vi "Read Value (variant).vi"(8 "error in (no error)":errorcluster, 11 "Bool D Element in":refnum<class "Bool D Element.lvclass">) -> (0 "error out":errorcluster, 2 "Variant":variant, 3 "Bool D Element out":refnum<class "Bool D Element.lvclass">)   [LabVIEW 2018, in "D Datagrid Library.lvlib" / "Bool D Element.lvclass"]
uses:
  Bool D Element.lvclass
  Bool D Element.lvclass/Bool D Element.ctl
  Read Value.vi
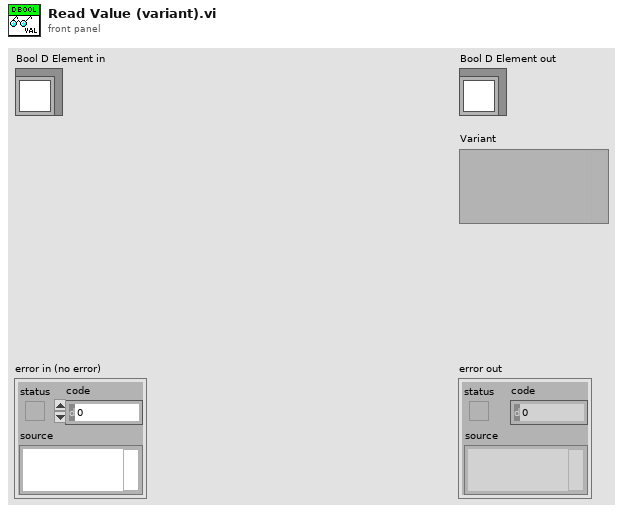
[diagram p1: front panel]
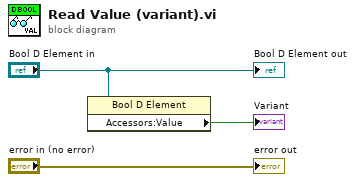
[diagram p0: block diagram]
diagram:
  n1 = property class="Bool D Element"(reference="Bool D Element in") -> ("Accessors:Value"=→"Variant":bool)  [unwired: 1 in, 2 out]
  "error out" <- "error in (no error)"
  "Bool D Element out" <- "Bool D Element in"
